vi "Format Step Size Data.vi"(0 "Max Frequency (Hz)":dbl format="%#_13g", 5 "Min Frequency (Hz)":dbl format="%#_13g", 11 "error in (no error)":errorcluster) -> (4 "Frequency[]":dbl[](array[numeric]) format="%#_6p", 15 "error out":errorcluster)   [LabVIEW 2020, in "LDO PSRR.lvlib"]
uses:
  LDO PSRR.lvlib
  256f91a7-304e-4e42-80fb-09493377d0e1.vi
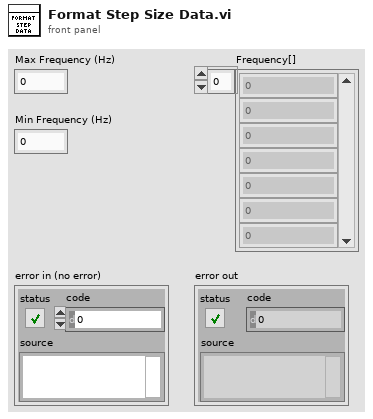
[diagram p1: front panel]
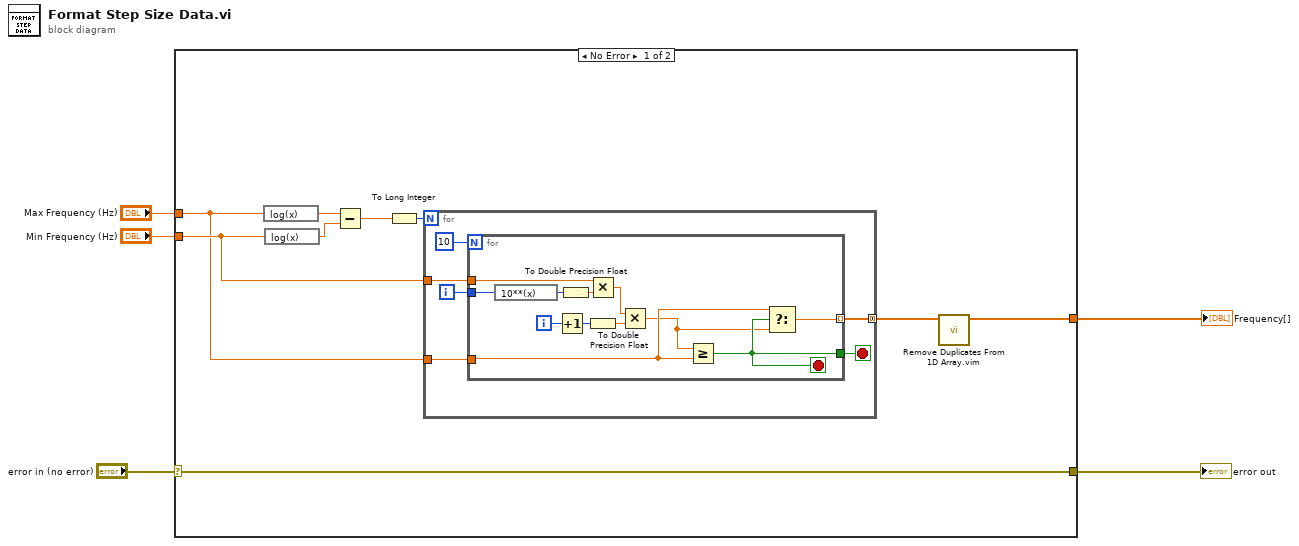
[diagram p0: block diagram]
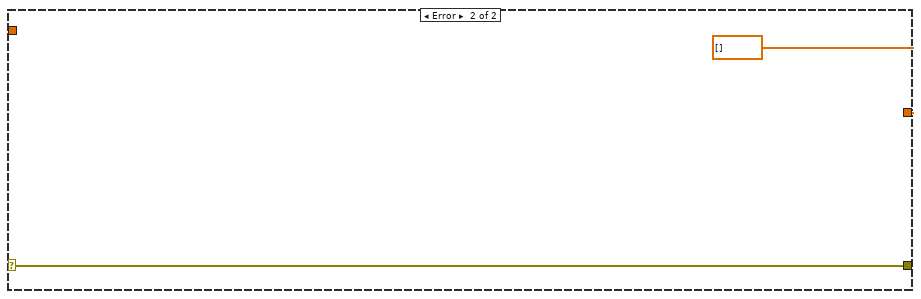
[diagram p2: hidden frame]
diagram:
  n1 = case shown="No Error" "error in (no error)" {
    selector: "error in (no error)" -> [w14 w34]
    tunnel: "Max Frequency (Hz)" -> [w9 _]
    tunnel: "Min Frequency (Hz)" -> [w11 _]
    tunnel: [w6 dbl[] []] -> w3
    tunnel: [w14 w34] -> w1
    frame No Error {
      n2 = expression code="log(x)"(w9) -> (w13:dbl)
      n3 = expression code="log(x)"(w11) -> (w12:dbl)
      n4 = Subtract(x=w13, y=w12) -> (x-y=w8:dbl)
      n5 = To Long Integer(number=w8) -> (32bit integer=w10:i32)
      n6 = for {
        N: w10 -> [_]
        tunnel: [w20] -> w7 mode=concatenating
        tunnel: w11 -> [w17]
        tunnel: w9 -> [w16]
        i -> [w18]
        stop <- w15 stop-if-true
        n7 = for {
          N: 10 -> [_]
          tunnel: w18 -> [w31]
          tunnel: [w24] -> w20 mode=indexing
          tunnel: w17 -> [w27]
          tunnel: w16 -> [w22]
          tunnel: [w23] -> w15
          i -> [w32]
          stop <- w23 stop-if-true
          n8 = expression code="10**(x)"(w31) -> (w28:i32)
          n9 = Increment(x=w32) -> (x+1=w30:i32)
          n10 = To Double Precision Float(number=w28) -> (double precision float=w26:dbl)
          n11 = Multiply(x=w27, y=w26) -> (x*y=w29:dbl)
          n12 = To Double Precision Float(number=w30) -> (double precision float=w25:dbl)
          n13 = Multiply(x=w29, y=w25) -> (x*y=w21:dbl)
          n14 = Greater Or Equal?(x=w21, y=w22) -> (x >= y?=w23:bool)
          n15 = Select(t=w22, s=w23, f=w21) -> (s? t:f=w24:dbl)
        }
      }
      n16 = call "Remove Duplicates From 1D Array.vim"("array"=w7) -> ("array with duplicates removed"=w6:dbl[])  [unwired: 10 in]
    }
    frame Error {
    }
  }
  "Frequency[]" <- w3
  "error out" <- w1
